vi "Parent_Create.vi"(0 "reference in":refnum<class "Parent.lvclass">, 5 "error in (no error)":errorcluster) -> (14 "reference out":refnum<class "Parent.lvclass">, 19 "error out":errorcluster)   [LabVIEW 2019, in "Parent.lvclass"]
uses:
  Parent.lvclass
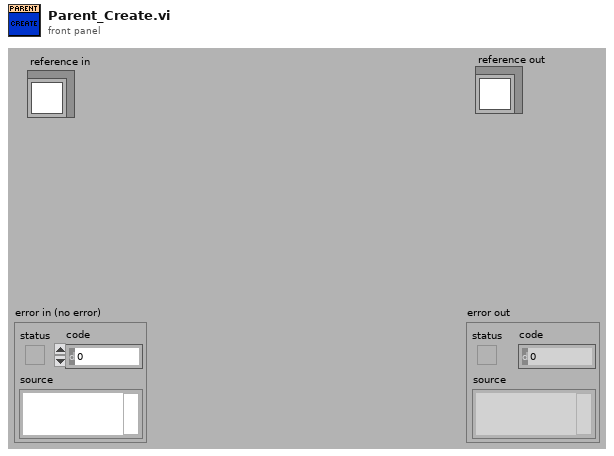
[diagram p1: front panel]
types:
  T1 = typedef "Parent.lvclass/ObjectAttributes.ctl" = cluster{"ParentAttribute":dbl}
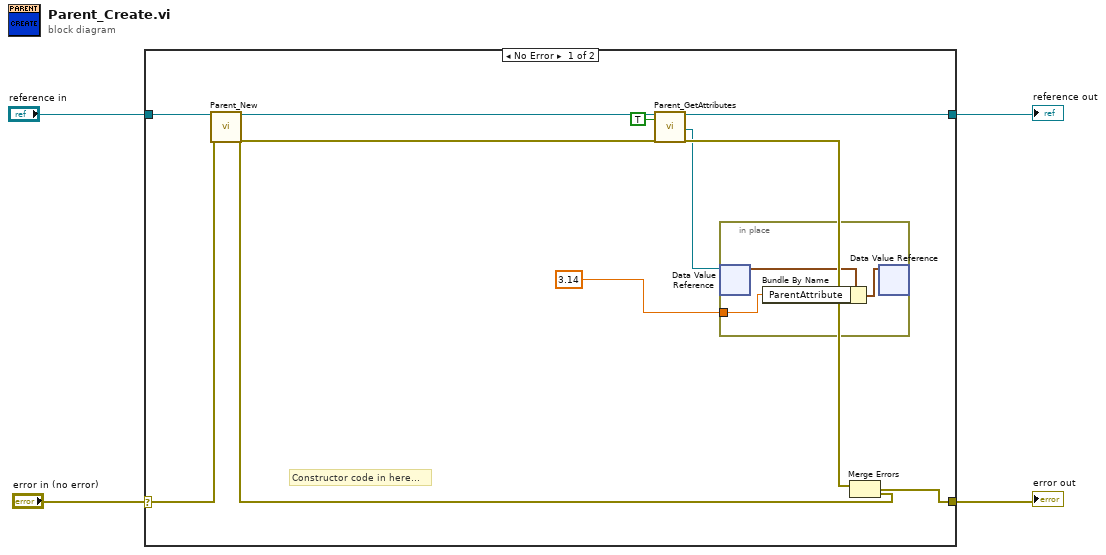
[diagram p0: block diagram]
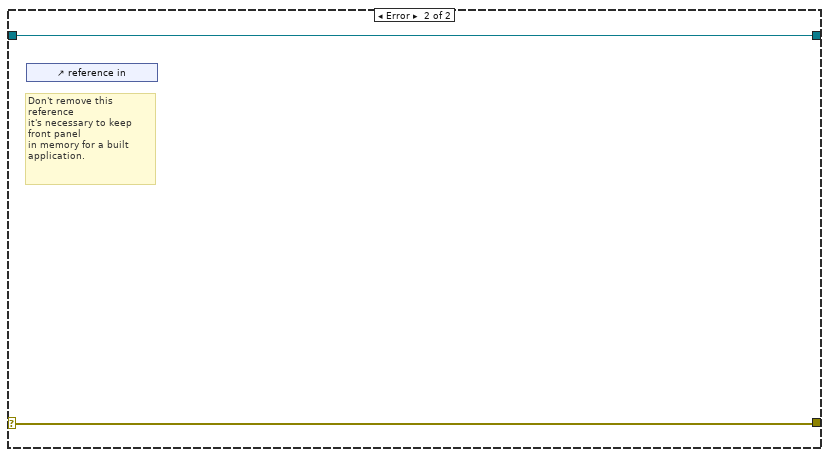
[diagram p2: hidden frame]
diagram:
  n1 = case shown="No Error" "error in (no error)" {
    selector: "error in (no error)" -> [w14 w19]
    tunnel: [w10 w19] -> w4
    tunnel: "reference in" -> [w12 w18]
    tunnel: [w13 w18] -> w2
    frame No Error {
      # "Constructor code in here..."
      n2 = call "Parent_New.vi"("reference in"=w12, "error in (no error)"=w14) -> ("reference out"=w11:refnum<class "Parent.lvclass">, "error out"=w8:errorcluster)  [unwired: 14 in, 2 out]
      n3 = call "Parent_GetAttributes.vi"("reference in"=w11, "OnlyGetDvrReference(False)"=TRUE, "error in (no error)"=w8) -> ("reference out"=w13:refnum<class "Parent.lvclass">, "DataRef"=w6:refnum<data-value>, "error out"=w9:errorcluster)  [unwired: 13 in, 1 out]
      n4 = in-place {
        in-place-border: 3.14 ("attribute1") -> [w16]
        n5 = in-place-dvr #1(w6) -> (w17:T1)  [unwired: 1 out]
        n6 = Bundle By Name(cluster=w17, "ParentAttribute"=w16) -> (w15:T1)
        n7 = in-place-dvr #1(w15) -> ()  [unwired: 2 out]
      }
      n8 = Merge Errors(w9, w8) -> (w10:errorcluster)
    }
    frame Error {
      # "Don't remove this reference\nit's necessary to keep front panel\nin memory for a built application."
      n9 = control-ref of="reference in"() -> ()  [unwired: 1 out]
    }
  }
  "error out" <- w4
  "reference out" <- w2
